vi "GA Pt Data.vi"(7 "dDataID":dbl, 8 "error in (no error)":errorcluster caption="错误输入（无错误）", 9 "lLength":i32, 10 "pData":i16, 11 "nAxisNum":i16) -> (0 "error out":errorcluster caption="错误输出", 2 "pData out":i16, 3 "function return":i32)   [LabVIEW 2015, in "GAS.lvlib"]
doc: "extern \"C\" __declspec(dllimport) int GA_PtData(short nAxisNum,short* pData,long lLength,double dDataID);"
uses:
  <userlib>/BP_GAS/GAS.lvlib
  <userlib>/BP_GAS/GAS.dll
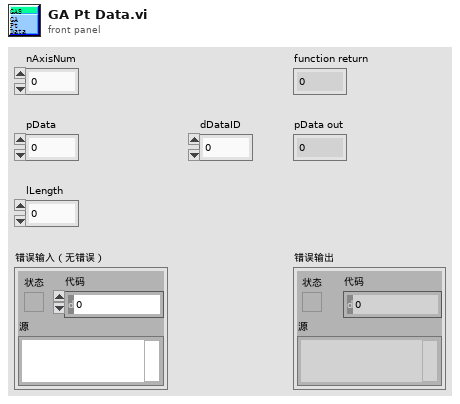
[diagram p1: front panel]
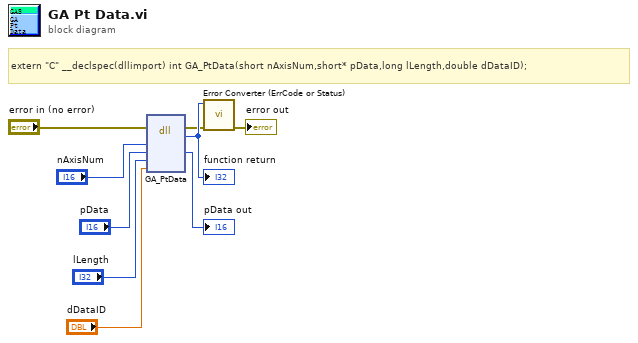
[diagram p0: block diagram]
diagram:
  # "extern \"C\" __declspec(dllimport) int GA_PtData(short nAxisNum,short* pData,long lLength,double dDataID);"
  n1 = dll-call lib="E:/Program Files (x86)/National Instruments/LabVIEW 2015/user.lib/BP_GAS/GAS.*" fn="GA_PtData"(error in="error in (no error)", "nAxisNum"="nAxisNum", "pData"="pData", "lLength"="lLength", "dDataID"="dDataID") -> (error out=w2:errorcluster, w9:i32, "pData"=→"pData out":i16)  [unwired: 5 in, 1 out]
  "function return" <- w9
  n2 = call "Error Converter (ErrCode or Status).vi"("error in (no error)"=w2, "error code"=w9) -> ("error out"=→"error out":errorcluster)  [unwired: 9 in]
